vi "GDSIconEditor_ImageDataTo8Bit.vi"(11 "image data":T1) -> (0 "NoMaskFound":bool, 1 "ColorArray":u32[](array[numeric]), 2 "8-bit pixmap":u8[][](array[numeric]), 3 "mask":u8[](array[numeric]) format="%08b")   [LabVIEW 2016]
uses:
  <vilib>/picture/picture.llb/imagedata.ctl
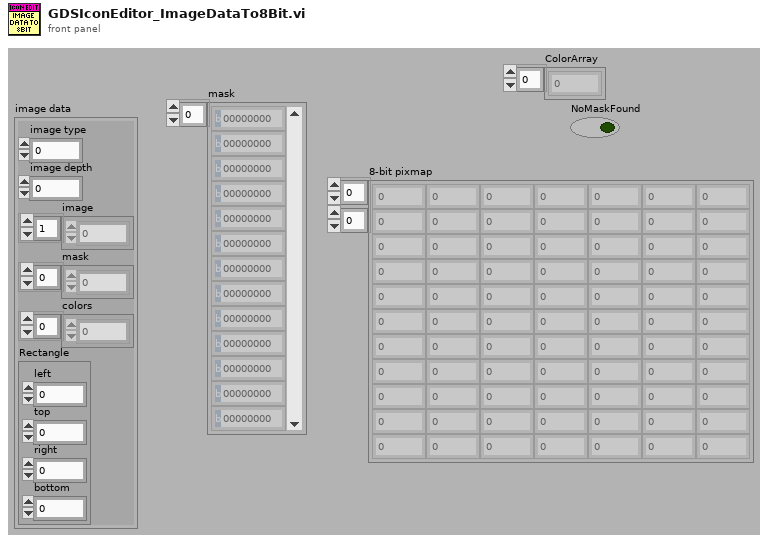
[diagram p1: front panel]
types:
  T1 = typedef "imagedata.ctl" = cluster{"image type":i32, "image depth":i32, "image":u8[], "mask":u8[], "colors":u32[], "Rectangle":cluster{"left":i16, "top":i16, "right":i16, "bottom":i16}}
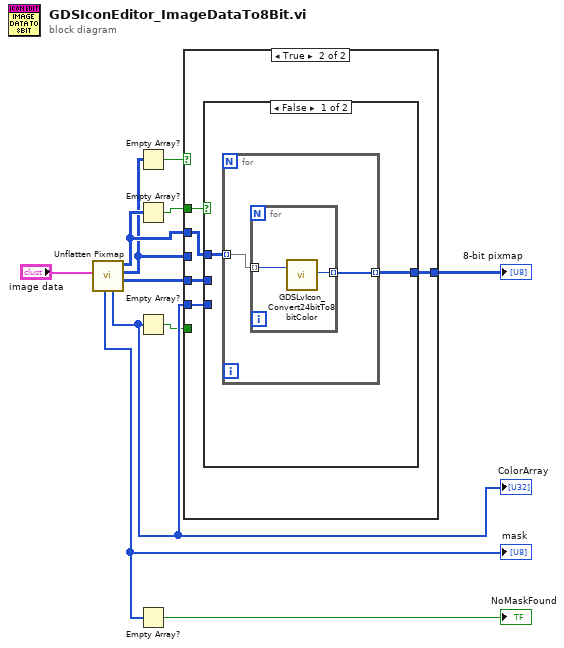
[diagram p0: block diagram]
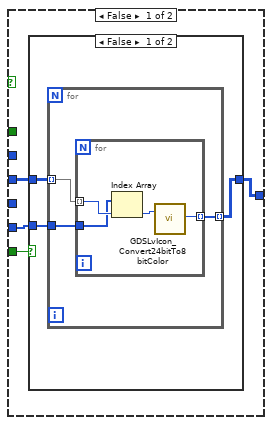
[diagram p2: hidden frame]
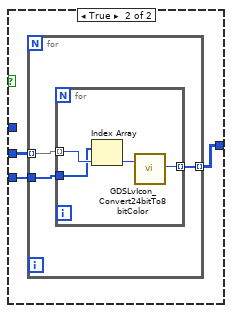
[diagram p4: hidden frame]
diagram:
  n1 = call <vilib>:"Unflatten Pixmap.vi"("image data"="image data") -> ("4-bit pixmap"=w9:u8[][], "8-bit pixmap"=w2:u8[][], "24-bit pixmap"=w10:u32[][], "colors"=w7:u32[], "mask"=w4:u8[])  [unwired: 4 in, 2 out]
  "ColorArray" <- w7
  "mask" <- w4
  n2 = Empty Array?(array=w2) -> (empty?=w1:bool)
  n3 = Empty Array?(array=w10) -> (empty?=w11:bool)
  n4 = Empty Array?(array=w7) -> (empty?=w6:bool)
  n5 = Empty Array?(array=w4) -> (empty?=→"NoMaskFound":bool)
  n6 = case shown="True" w1 {
    tunnel: w10 -> [_ w31]
    tunnel: w2 -> [w14 _]
    tunnel: [w13 w30] -> w8
    tunnel: w6 -> [w15 _]
    tunnel: w7 -> [w12 w28]
    tunnel: w9 -> [_ w27]
    tunnel: w11 -> [_ w29]
    frame False {
      n7 = case shown="False" w15 {
        tunnel: w14 -> [w18 w26]
        tunnel: [w16 w26] -> w13
        tunnel: w12 -> [w17 _]
        frame False {
          n8 = for {
            tunnel: w18 -> [w21] mode=indexing
            tunnel: w17 -> [w20]
            tunnel: [w19] -> w16 mode=indexing
            n9 = for {
              tunnel: w21 -> [w25] mode=indexing
              tunnel: w20 -> [w24]
              tunnel: [w22] -> w19 mode=indexing
              n10 = Index Array(array=w24, index=w25) -> (element=w23:u32)
              n11 = call <resource>:"GDSLvIcon_Convert24bitTo8bitColor.vi"("Color 24bit In"=w23) -> ("Color out(256)"=w22:u8)  [unwired: 15 in, 3 out]
            }
          }
        }
        frame True {
        }
      }
    }
    frame True {
      n12 = case shown="False" w29 {
        tunnel: w31 -> [w33 _]
        tunnel: [w32 w39] -> w30
        tunnel: w28 -> [_ w40]
        tunnel: w27 -> [_ w38]
        frame False {
          n13 = for {
            tunnel: w33 -> [w35] mode=indexing
            tunnel: [w34] -> w32 mode=indexing
            n14 = for {
              tunnel: w35 -> [w37] mode=indexing
              tunnel: [w36] -> w34 mode=indexing
              n15 = call <resource>:"GDSLvIcon_Convert24bitTo8bitColor.vi"("Color 24bit In"=w37) -> ("Color out(256)"=w36:u8)  [unwired: 15 in, 3 out]
            }
          }
        }
        frame True {
          n16 = for {
            tunnel: w38 -> [w43] mode=indexing
            tunnel: w40 -> [w42]
            tunnel: [w41] -> w39 mode=indexing
            n17 = for {
              tunnel: w43 -> [w47] mode=indexing
              tunnel: w42 -> [w46]
              tunnel: [w44] -> w41 mode=indexing
              n18 = Index Array(array=w46, index=w47) -> (element=w45:u32)
              n19 = call <resource>:"GDSLvIcon_Convert24bitTo8bitColor.vi"("Color 24bit In"=w45) -> ("Color out(256)"=w44:u8)  [unwired: 15 in, 3 out]
            }
          }
        }
      }
    }
  }
  "8-bit pixmap" <- w8
